vi "Finish.vi"   [LabVIEW 2011]
doc: "This VI is called just before exiting. It is expected to close I/O refnum, save collected data, etc."
uses:
  <vilib>/Rock Robotics/WPI/Compressor/WPI_CompressorGetSetRefNum.vi
types:
  T1 = typedef "WPI_RobotDriveDevRef.ctl" = cluster{"DevStatus":errorcluster, "Motors[]":T2[], "Square Inputs":bool, "Max Output":dbl, "Isochronous":bool}
  T2 = typedef "WPI_MotorControlDeviceRef.ctl" = cluster{"DeviceStatus":errorcluster, "Type":enum16{"PWM", "CAN"}, "PWM":cluster{"Digital Module":T3, "PWM Channel":T4, "DeadBand":T5}, "CAN":cluster{"Device Number":u8, "Control Mode":T6, "Semaphore":T7, "Max Vout":dbl}, "Invert":bool, "TransformRef":T8, "InvTransformRef":T8}
  T3 = typedef "FPGA_TypedefDigitalModule.ctl" = enum16{"Digital Module 1", "Digital Module 2"}
  T4 = typedef "FPGA_DIOPWMChannel.ctl" = enum8{"PWM 1", "PWM 2", "PWM 3", "PWM 4", "PWM 5", "PWM 6", "PWM 7", "PWM 8", "PWM 9", "PWM 10", "Invalid"}
  T5 = typedef "WPI_PWMDeadband.ctl" = cluster{"Name":string, "maxPositivePwm":i32, "minPositivePwm":i32, "centerPwm":i32, "maxNegativePwm":i32, "minNegativePwm":i32, "angularRange":u16}
  T6 = typedef "WPI_CANJaguar_ControlMode.ctl" = enum8{"Percent VBus", "Current", "Speed", "Position", "Voltage"}
  T7 = typedef "Semaphore RefNum" = refnum<k1>
  T8 = typedef "WPI_PWMTransform_ConPane.ctl" = refnum<vi>
  T9 = typedef "WPI_SolenoidDevRef.ctl" = cluster{"DevStatus":errorcluster, "Solenoid Module":T10, "Forward Solenoid Channel":T11, "Reverse Solenoid Channel":T11}
  T10 = typedef "FPGA_TypedefSolenoidModule.ctl" = enum16{"Solenoid Module 1", "Solenoid Module 2"}
  T11 = typedef "WPI_SolenoidChannel.ctl" = enum8{"Solenoid 1", "Solenoid 2", "Solenoid 3", "Solenoid 4", "Solenoid 5", "Solenoid 6", "Solenoid 7", "Solenoid 8", "Invalid"}
  T12 = typedef "WPI_CompressorDevRef.ctl" = cluster{"DevStatus":errorcluster, "DigitalInputDevRef":T13, "RelayDevRef":T15}
  T13 = typedef "WPI_DigitalInputDevRef.ctl" = cluster{"DevStatus":errorcluster, "DIO Channel":T14, "Digital Module":T3}
  T14 = typedef "FPGA_DIOChannel.ctl" = enum8{"DIO 1", "DIO 2", "DIO 3", "DIO 4", "DIO 5", "DIO 6", "DIO 7", "DIO 8", "DIO 9", "DIO 10", "DIO 11", "DIO 12", "DIO 13", "DIO 14", "Invalid"}
  T15 = typedef "WPI_RelayDevRef.ctl" = cluster{"DevStatus":errorcluster, "Relay Channel":T16, "Digital Module":T3, "Relay Direction":T17}
  T16 = typedef "FPGA_DIORelayChannel.ctl" = enum8{"Relay 1", "Relay 2", "Relay 3", "Relay 4", "Relay 5", "Relay 6", "Relay 7", "Relay 8", "Invalid"}
  T17 = typedef "WPI_RelayDirection.ctl" = enum16{"Both directions", "Forward only", "Reverse only"}
  T18 = typedef "WPI_DigitalOutputDevRef.ctl" = cluster{"Digital Module":T3, "DIO Channel":T14, "DevStatus":errorcluster}
  T19 = typedef "WPI_JoystickDevRef.ctl" = cluster{"Device":T20}
  T20 = typedef "WPI_JoystickDeviceEnum.ctl" = enum16{"USB 1", "USB 2", "USB 3", "USB 4", "Kinect 1", "Kinect 2"}
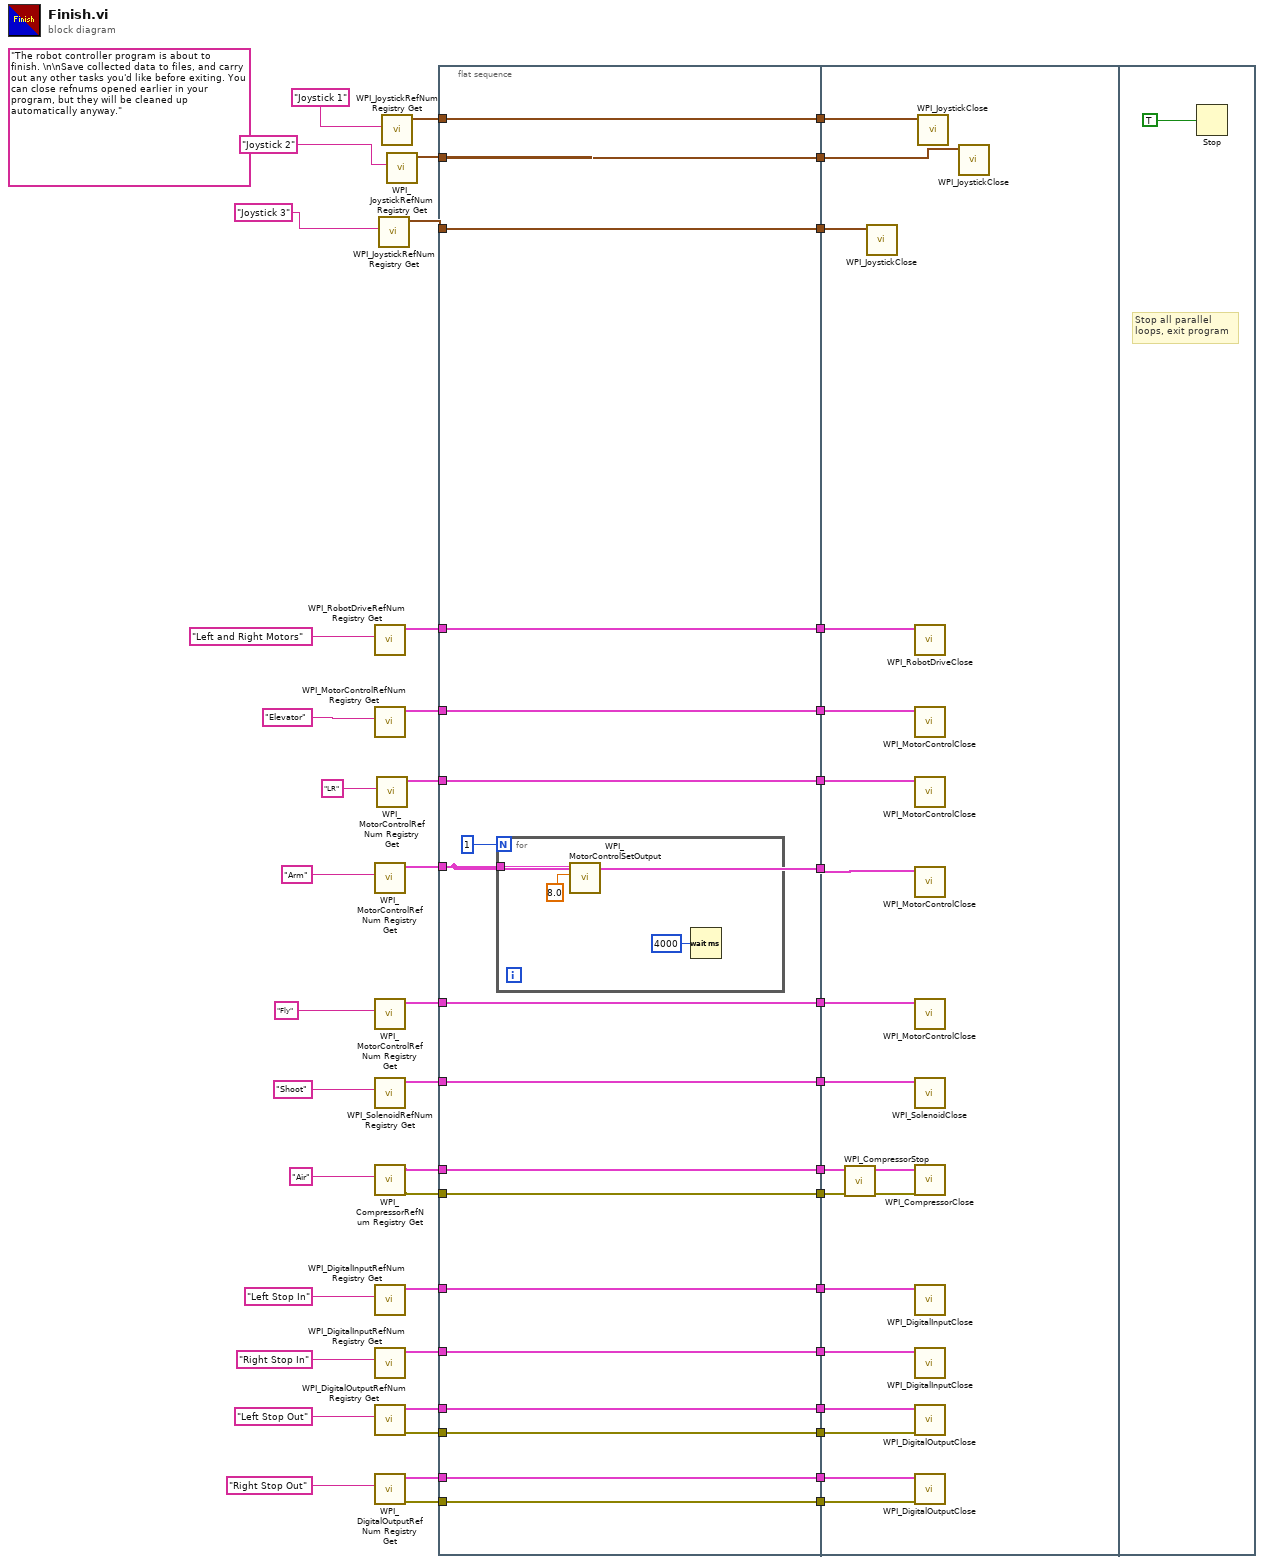
[diagram p0: block diagram]
diagram:
  (unwired) "The robot controller program is about to finish. \n\nSave collected data to files, and carry out any other tasks you'd like before exiting. You can close refnums opened earlier in your program, but they will be cleaned up automatically anyway."
  n1 = call <vilib>:"WPI_RobotDriveRefNum Registry Get.vi"("refnum name"="Left and Right Motors") -> ("RobotDriveDevRef"=w46:T1)  [unwired: 1 in, 9 out]
  n2 = call <vilib>:"WPI_MotorControlRefNum Registry Get.vi"("refnum name"="Elevator") -> ("MotorControlDevRef"=w40:T2)  [unwired: 9 in, 1 out]
  n3 = call <vilib>:"WPI_MotorControlRefNum Registry Get.vi"("refnum name"="Arm") -> ("MotorControlDevRef"=w38:T2)  [unwired: 9 in, 1 out]
  n4 = call <vilib>:"WPI_MotorControlRefNum Registry Get.vi"("refnum name"="Fly") -> ("MotorControlDevRef"=w37:T2)  [unwired: 9 in, 1 out]
  n5 = call <vilib>:"WPI_SolenoidRefNum Registry Get.vi"("refnum name"="Shoot") -> ("SolenoidDevRef"=w36:T9)  [unwired: 9 in, 1 out]
  n6 = call <vilib>:"WPI_CompressorRefNum Registry Get.vi"("refnum name"="Air") -> ("error out"=w34:errorcluster, "CompressorDevRef"=w35:T12)  [unwired: 9 in]
  n7 = call <vilib>:"WPI_DigitalInputRefNum Registry Get.vi"("refnum name"="Left Stop In") -> ("DigitalInputDevRef"=w33:T13)  [unwired: 9 in, 1 out]
  n8 = call <vilib>:"WPI_DigitalInputRefNum Registry Get.vi"("refnum name"="Right Stop In") -> ("DigitalInputDevRef"=w32:T13)  [unwired: 9 in, 1 out]
  n9 = call <vilib>:"WPI_DigitalOutputRefNum Registry Get.vi"("refnum name"="Left Stop Out") -> ("error out"=w9:errorcluster, "DigitalOutputDevRef"=w11:T18)  [unwired: 9 in]
  n10 = call <vilib>:"WPI_DigitalOutputRefNum Registry Get.vi"("refnum name"="Right Stop Out") -> ("error out"=w8:errorcluster, "DigitalOutputDevRef"=w6:T18)  [unwired: 9 in]
  n11 = call <vilib>:"WPI_MotorControlRefNum Registry Get.vi"("refnum name"="LR") -> ("MotorControlDevRef"=w39:T2)  [unwired: 9 in, 1 out]
  n12 = call <vilib>:"WPI_JoystickRefNum Registry Get.vi"("refnum name"="Joystick 3") -> ("JoystickDevRef"=w41:T19)  [unwired: 9 in, 1 out]
  n13 = call <vilib>:"WPI_JoystickRefNum Registry Get.vi"("refnum name"="Joystick 1") -> ("JoystickDevRef"=w45:T19)  [unwired: 1 in, 9 out]
  n14 = call <vilib>:"WPI_JoystickRefNum Registry Get.vi"("refnum name"="Joystick 2") -> ("JoystickDevRef"=w44:T19)  [unwired: 9 in, 1 out]
  n15 = flat-sequence {
    tunnel: w32 -> [w55]
    tunnel: w33 -> [w56]
    tunnel: w34 -> [w57]
    tunnel: w35 -> [w58]
    tunnel: w36 -> [w59]
    tunnel: w37 -> [w60]
    tunnel: w38 -> [w54]
    tunnel: w39 -> [w61]
    tunnel: w40 -> [w62]
    tunnel: w41 -> [w63]
    tunnel: w44 -> [w64]
    tunnel: w45 -> [w65]
    tunnel: w46 -> [w66]
    tunnel: [w66] -> w31
    tunnel: [w65] -> w30
    tunnel: [w64] -> w29
    tunnel: [w63] -> w28
    tunnel: [w62] -> w27
    tunnel: [w61] -> w26
    tunnel: [w60] -> w25
    tunnel: [w59] -> w24
    tunnel: [w58] -> w23
    tunnel: [w57] -> w22
    tunnel: [w56] -> w21
    tunnel: [w55] -> w20
    tunnel: [w54] -> w19
    tunnel: [w53] -> w12
    tunnel: w11 -> [w53]
    tunnel: [w52] -> w10
    tunnel: w9 -> [w52]
    tunnel: w8 -> [w51]
    tunnel: [w51] -> w7
    tunnel: w6 -> [w50]
    tunnel: [w50] -> w5
    tunnel: w31 -> [w88]
    tunnel: w30 -> [w87]
    tunnel: w29 -> [w86]
    tunnel: w28 -> [w85]
    tunnel: w27 -> [w84]
    tunnel: w26 -> [w83]
    tunnel: w25 -> [w82]
    tunnel: w24 -> [w81]
    tunnel: w23 -> [w80]
    tunnel: w22 -> [w79]
    tunnel: w21 -> [w78]
    tunnel: w20 -> [w77]
    tunnel: w19 -> [w76]
    tunnel: w12 -> [w73]
    tunnel: w10 -> [w72]
    tunnel: w7 -> [w71]
    tunnel: w5 -> [w70]
    frame #0 {
      n16 = for {
        N: 1 -> [_]
        tunnel: w54 -> [w69]
        n17 = call <vilib>:"WPI_MotorControlSetOutput.vi"("Output"=8.0, "MotorControlDevRef"=w69) -> ()  [unwired: 8 in, 2 out]
        n18 = Wait (ms)(milliseconds to wait=u32 4000) -> ()  [unwired: 1 out]
      }
    }
    frame #1 {
      n19 = call <vilib>:"WPI_CompressorStop.vi"("error in (no error)"=w79, "CompressorDevRef"=w80) -> ("error out"=w75:errorcluster, "CompressorDevRef"=w74:T12)  [unwired: 8 in]
      n20 = call <vilib>:"WPI_JoystickClose.vi"("JoystickDevRef"=w85) -> ()  [unwired: 11 in]
      n21 = call <vilib>:"WPI_RobotDriveClose.vi"("RobotDriveDevRef"=w88) -> ()  [unwired: 1 in, 10 out]
      n22 = call <vilib>:"WPI_MotorControlClose.vi"("MotorControlDevRef"=w84) -> ()  [unwired: 10 in, 1 out]
      n23 = call <vilib>:"WPI_MotorControlClose.vi"("MotorControlDevRef"=w83) -> ()  [unwired: 10 in, 1 out]
      n24 = call <vilib>:"WPI_MotorControlClose.vi"("MotorControlDevRef"=w76) -> ()  [unwired: 10 in, 1 out]
      n25 = call <vilib>:"WPI_MotorControlClose.vi"("MotorControlDevRef"=w82) -> ()  [unwired: 10 in, 1 out]
      n26 = call <vilib>:"WPI_SolenoidClose.vi"("SolenoidDevRef"=w81) -> ()  [unwired: 10 in, 1 out]
      n27 = call <vilib>:"WPI_CompressorClose.vi"("error in (no error)"=w75, "CompressorDevRef"=w74) -> ()  [unwired: 9 in, 1 out]
      n28 = call <vilib>:"WPI_DigitalInputClose.vi"("DigitalInputDevRef"=w78) -> ()  [unwired: 10 in, 1 out]
      n29 = call <vilib>:"WPI_DigitalInputClose.vi"("DigitalInputDevRef"=w77) -> ()  [unwired: 10 in, 1 out]
      n30 = call <vilib>:"WPI_DigitalOutputClose.vi"("error in (no error)"=w72, "DigitalOutputDevRef"=w73) -> ()  [unwired: 9 in, 1 out]
      n31 = call <vilib>:"WPI_DigitalOutputClose.vi"("error in (no error)"=w71, "DigitalOutputDevRef"=w70) -> ()  [unwired: 9 in, 1 out]
      n32 = call <vilib>:"WPI_JoystickClose.vi"("JoystickDevRef"=w87) -> ()  [unwired: 11 out]
      n33 = call <vilib>:"WPI_JoystickClose.vi"("JoystickDevRef"=w86) -> ()  [unwired: 11 in]
    }
    frame #2 {
      # "Stop all parallel\nloops, exit program"
      n34 = Stop(stop? (T)=TRUE ("Quit")) -> ()
    }
  }
